vi "Update Deploying Dialog Box.vi"(8 "error in (no error)":errorcluster, 10 "Text to add":string, 11 "Details Ref in":refnum<vi>) -> (0 "error out":errorcluster, 3 "Details Ref out":refnum<vi>)   [LabVIEW 2019, in "Ballard Arinc-429 System Explorer.lvlib"]
uses:
  Ballard Arinc-429 System Explorer.lvlib
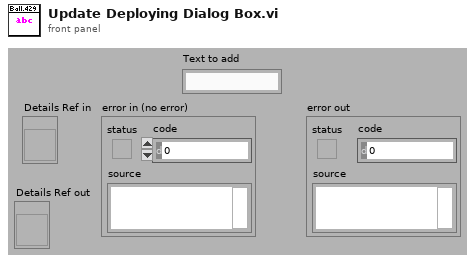
[diagram p1: front panel]
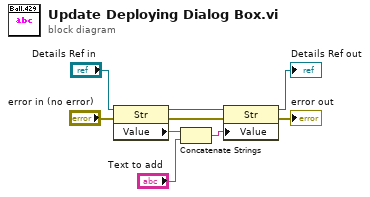
[diagram p0: block diagram]
diagram:
  n1 = property class="Str"(reference="Details Ref in", error in="error in (no error)") -> (reference out=w6:refnum<vi>, error out=w5:errorcluster, "Value"=w4:string)
  n2 = Concatenate Strings(w4, "Text to add") -> (w7:string)
  n3 = property class="Str"(reference=w6, error in=w5, "Value"=w7) -> (reference out=→"Details Ref out":refnum<vi>, error out=→"error out":errorcluster)
